vi "Calculator to solve.vi"() -> ()   [LabVIEW 2014]
panel:
  out "Result":dbl
  in  "?":bool
  in  "Number b":dbl
  in  "Number a":dbl
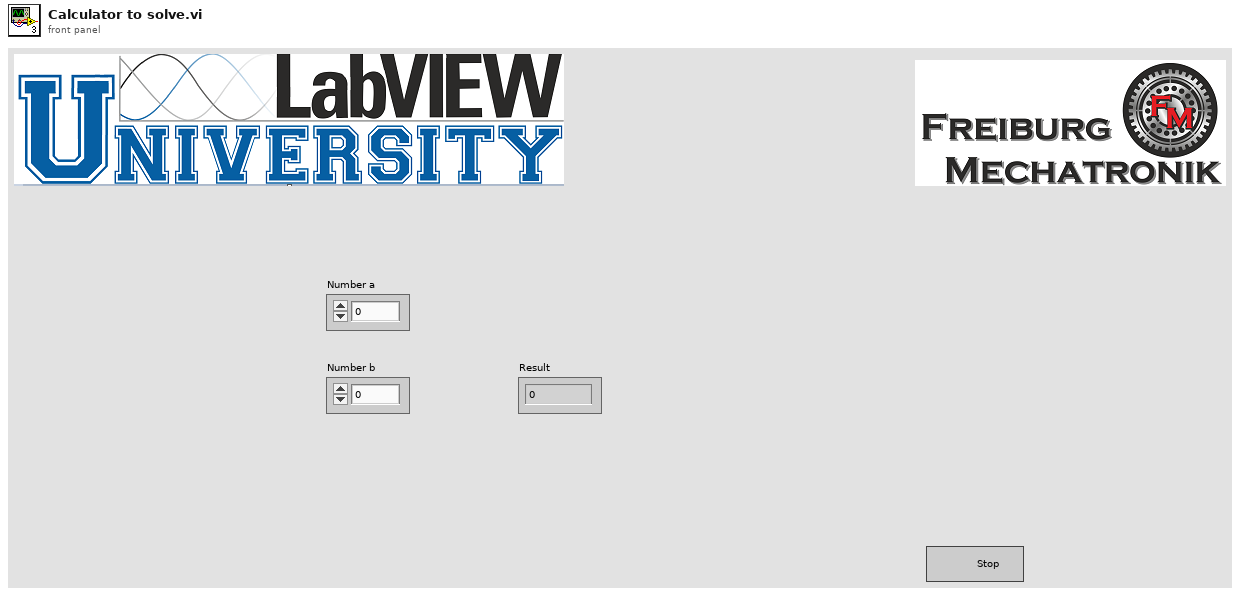
[diagram p1: front panel]
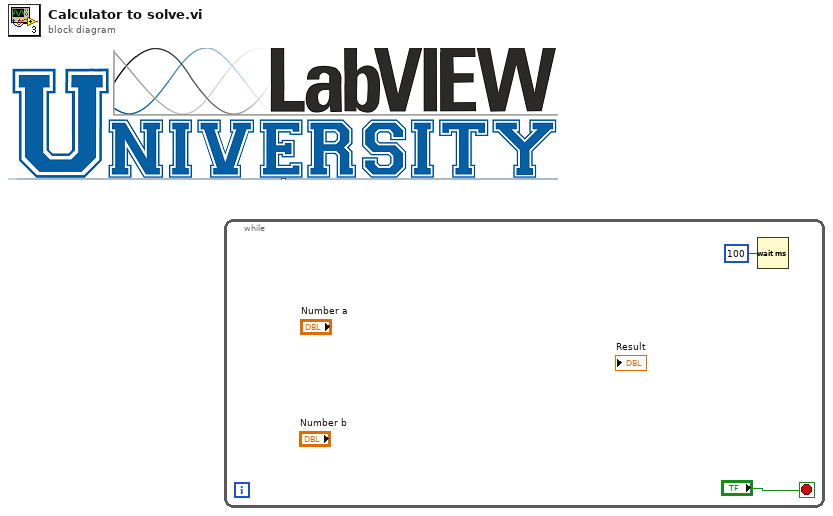
[diagram p0: block diagram]
diagram:
  n1 = while {
    stop <- "?" stop-if-true
    n2 = Wait (ms)(milliseconds to wait=u32 100) -> ()  [unwired: 1 out]
  }
